vi "Update display current.vi"(8 "error in (no error)":errorcluster, 11 "StageSPIM in":refnum<class "StageSPIM.lvclass">) -> (0 "error out":errorcluster, 3 "StageSPIM out":refnum<class "StageSPIM.lvclass">)   [LabVIEW 2012, in "StageSPIM.lvclass"]
uses:
  StageSPIM.lvclass
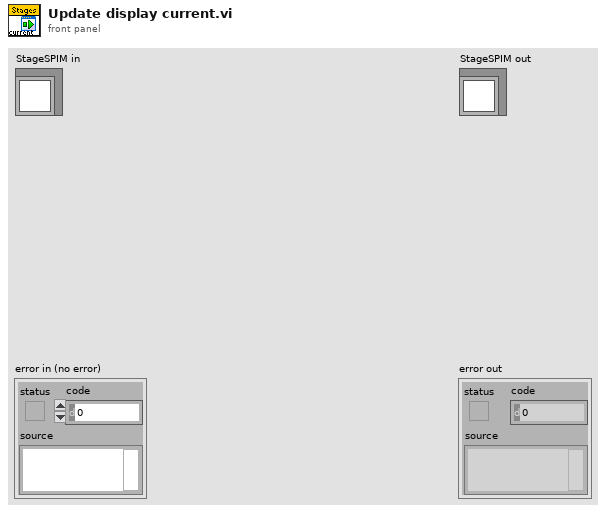
[diagram p1: front panel]
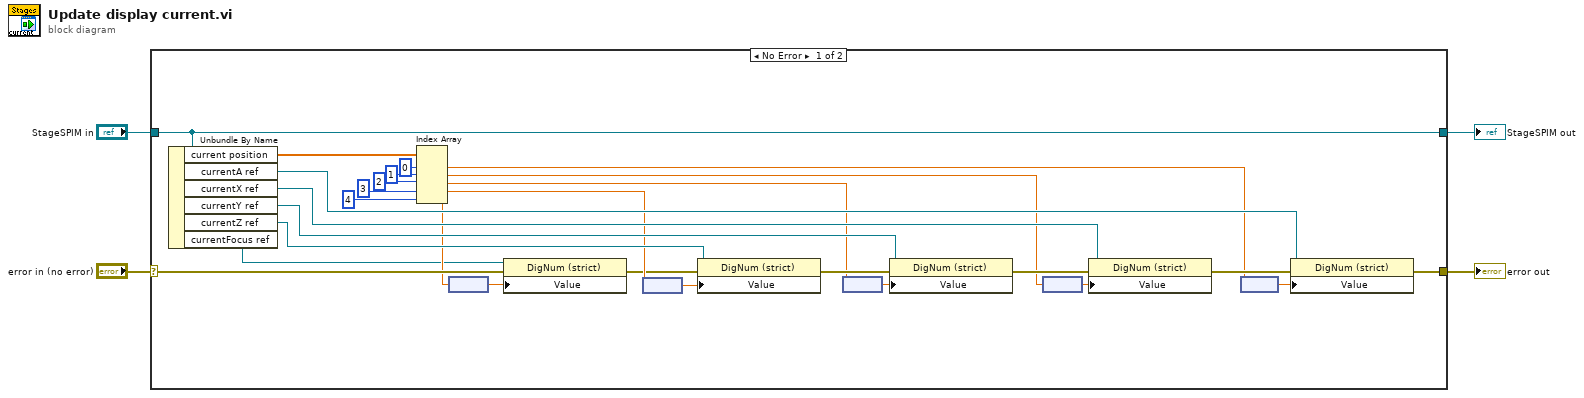
[diagram p0: block diagram]
diagram:
  n1 = case shown="No Error" "error in (no error)" {
    selector: "error in (no error)" -> [w8 w34]
    tunnel: [w19 w34] -> w3
    tunnel: [w32 w33] -> w1
    tunnel: "StageSPIM in" -> [w32 w33]
    frame No Error {
      n2 = Unbundle By Name(w32) -> ("current position"=w31:dbl[], "currentA ref"=w23:refnum<vi>, "currentX ref"=w24:refnum<vi>, "currentY ref"=w25:refnum<vi>, "currentZ ref"=w26:refnum<vi>, "currentFocus ref"=w5:refnum<vi>)
      n3 = Index Array(array=w31, index #1=0 ("index"), index #2=1 ("index"), index #3=2 ("index"), index #4=3 ("index"), index #5=4 ("index")) -> (element #1=w11:dbl, element #2=w13:dbl, element #3=w15:dbl, element #4=w17:dbl, element #5=w6:dbl)
      n4 = node(w6) -> (w9:dbl[unit])
      n5 = property class="DigNum (strict)"(reference=w5, error in=w8, "Value"=w9) -> (error out=w7:errorcluster)  [unwired: 1 out]
      n6 = node(w17) -> (w18:dbl[unit])
      n7 = property class="DigNum (strict)"(reference=w26, error in=w7, "Value"=w18) -> (error out=w22:errorcluster)  [unwired: 1 out]
      n8 = node(w15) -> (w16:dbl[unit])
      n9 = property class="DigNum (strict)"(reference=w25, error in=w22, "Value"=w16) -> (error out=w21:errorcluster)  [unwired: 1 out]
      n10 = node(w13) -> (w14:dbl[unit])
      n11 = property class="DigNum (strict)"(reference=w24, error in=w21, "Value"=w14) -> (error out=w20:errorcluster)  [unwired: 1 out]
      n12 = node(w11) -> (w12:dbl[unit])
      n13 = property class="DigNum (strict)"(reference=w23, error in=w20, "Value"=w12) -> (error out=w19:errorcluster)  [unwired: 1 out]
    }
    frame Error {
    }
  }
  "error out" <- w3
  "StageSPIM out" <- w1
